vi "Modbus to Float.vi"(10 "Registers":u16[](array[numeric])) -> (2 "32-Bit Float":sgl)   [LabVIEW 2024, in "Bronkhorst Flexi-Flow ModbusTCP API.lvlib"]
uses:
  Bronkhorst Flexi-Flow ModbusTCP API.lvlib
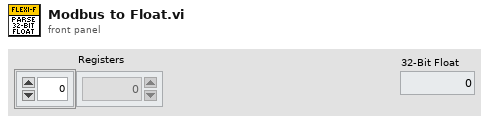
[diagram p1: front panel]
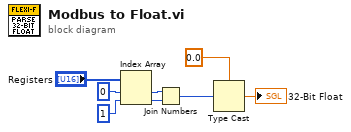
[diagram p0: block diagram]
diagram:
  n1 = Index Array(array="Registers", index #1=0 ("index"), index #2=1 ("index")) -> (element #1=w5:u16, element #2=w4:u16)
  n2 = Join Numbers(hi=w5, lo=w4) -> ((hi.lo)=w3:u32)
  n3 = Type Cast(type=sgl 0.0, x=w3) -> (*(type *) &x=→"32-Bit Float":sgl)
